vi "Preserve niDCPower Settings - PAE.vi"(7 "Action":enum16{"Reserve Settings", "Re-apply Settings"}(ring), 8 "error in":errorcluster, 10 "Active Channel":string="0", 11 "Resource Name":refnum<k15>="Dev1/0") -> (0 "error out":errorcluster, 1 "output cluster":T1, 2 "Active Channel":string="0", 3 "Resource Name":refnum<k15>)   [LabVIEW 2023]
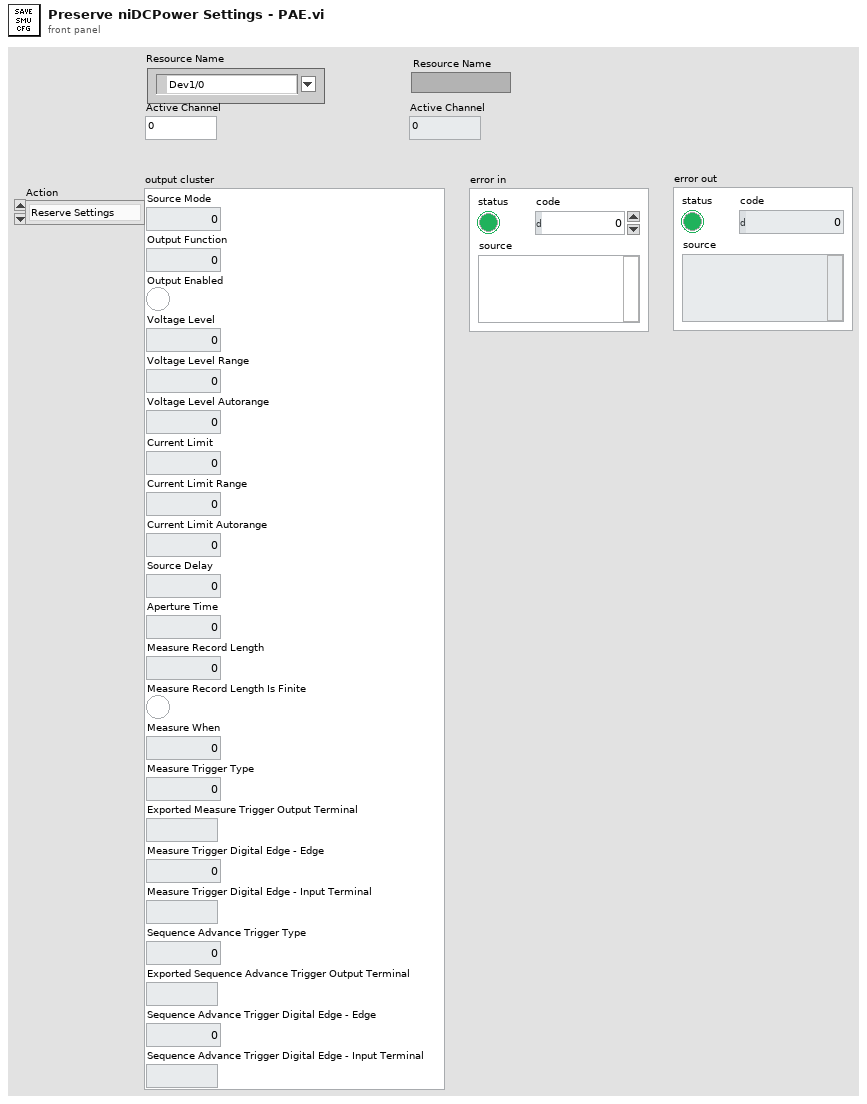
[diagram p1: front panel]
types:
  T1 = cluster{"Source Mode":i32, "Output Function":i32, "Output Enabled":bool, "Voltage Level":dbl, "Voltage Level Range":dbl, "Voltage Level Autorange":i32, "Current Limit":dbl, "Current Limit Range":dbl, "Current Limit Autorange":i32, "Source Delay":dbl, "Aperture Time":dbl, "Measure Record Length":i32, "Measure Record Length Is Finite":bool, "Measure When":i32, "Measure Trigger Type":i32, "Exported Measure Trigger Output Terminal":string, "Measure Trigger Digital Edge - Edge":i32, "Measure Trigger Digital Edge - Input Terminal":string, "Sequence Advance Trigger Type":i32, "Exported Sequence Advance Trigger Output Terminal":string, "Sequence Advance Trigger Digital Edge - Edge":i32, "Sequence Advance Trigger Digital Edge - Input Terminal":string}
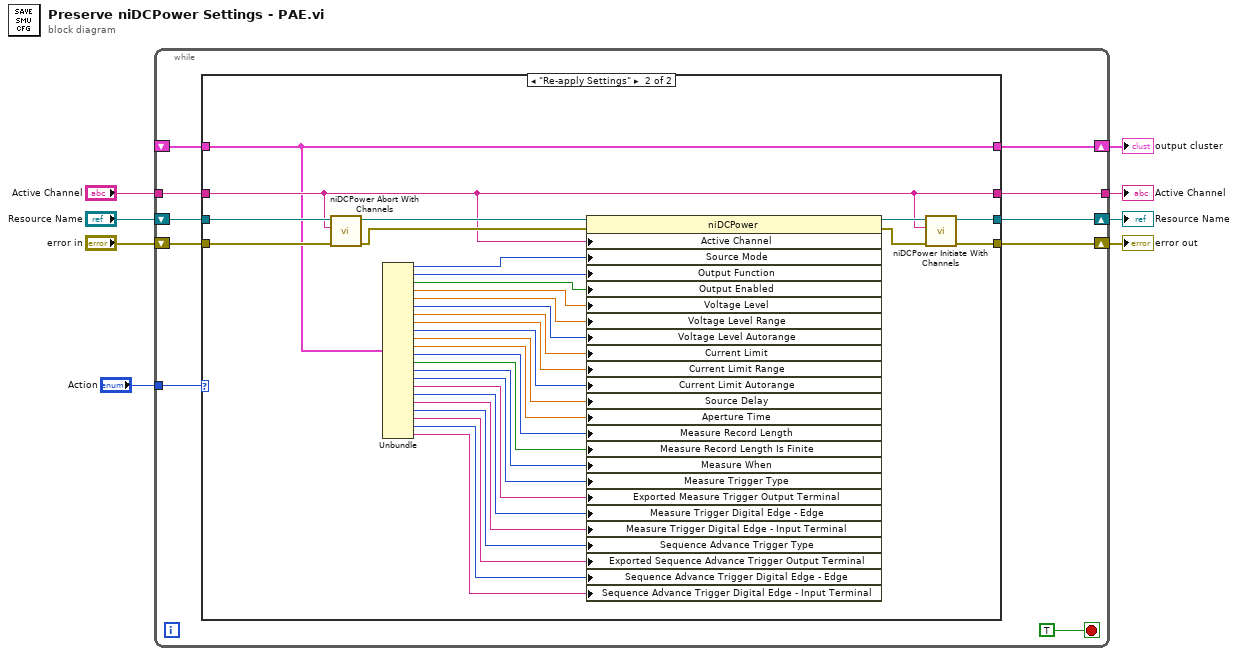
[diagram p0: block diagram]
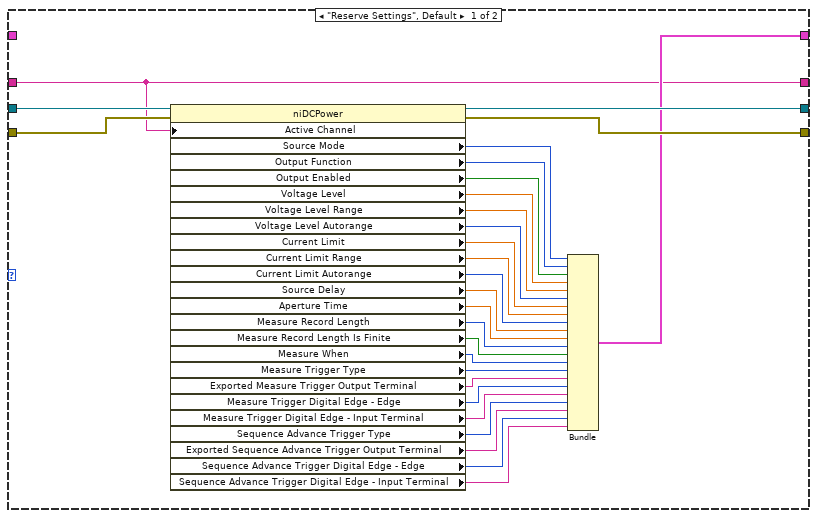
[diagram p2: hidden frame]
diagram:
  n1 = while {
    shift-right: [w16] -> w6
    shift-left: "Resource Name" -> [w18]
    shift-right: [w17] -> w7
    shift-left: "error in" -> [w15]
    shift-right: [w14] -> w1
    shift-left: _ -> [w12]
    tunnel: "Action" -> [w11]
    tunnel: "Active Channel" -> [w10]
    tunnel: [w9] -> w2
    stop <- TRUE stop-if-true
    n2 = case shown="\"Re-apply Settings\"" w11 {
      tunnel: w18 -> [w46 w56]
      tunnel: [w45 w51] -> w17
      tunnel: [w43 w49] -> w16
      tunnel: w15 -> [w21 w54]
      tunnel: [w20 w47] -> w14
      tunnel: w12 -> [_ w47]
      tunnel: w10 -> [w19 w48]
      tunnel: [w19 w48] -> w9
      frame "Reserve Settings", Default {
        n3 = property class="niDCPower"(reference=w46, error in=w21, "Active Channel"=w19) -> (reference out=w43:refnum<k15>, error out=w45:errorcluster, "Source Mode"=w44:i32, "Output Function"=w42:i32, "Output Enabled"=w41:bool, "Voltage Level"=w40:dbl, "Voltage Level Range"=w39:dbl, "Voltage Level Autorange"=w38:i32, "Current Limit"=w37:dbl, "Current Limit Range"=w36:dbl, "Current Limit Autorange"=w35:i32, "Source Delay"=w34:dbl, "Aperture Time"=w33:dbl, "Measure Record Length"=w32:i32, "Measure Record Length Is Finite"=w31:bool, "Measure When"=w30:i32, "Measure Trigger Type"=w29:i32, "Exported Measure Trigger Output Terminal"=w28:string, "Measure Trigger Digital Edge - Edge"=w27:i32, "Measure Trigger Digital Edge - Input Terminal"=w26:string, "Sequence Advance Trigger Type"=w25:i32, "Exported Sequence Advance Trigger Output Terminal"=w24:string, "Sequence Advance Trigger Digital Edge - Edge"=w23:i32, "Sequence Advance Trigger Digital Edge - Input Terminal"=w22:string)
        n4 = Bundle("Source Mode"=w44, "Output Function"=w42, "Output Enabled"=w41, "Voltage Level"=w40, "Voltage Level Range"=w39, "Voltage Level Autorange"=w38, "Current Limit"=w37, "Current Limit Range"=w36, "Current Limit Autorange"=w35, "Source Delay"=w34, "Aperture Time"=w33, "Measure Record Length"=w32, "Measure Record Length Is Finite"=w31, "Measure When"=w30, "Measure Trigger Type"=w29, "Exported Measure Trigger Output Terminal"=w28, "Measure Trigger Digital Edge - Edge"=w27, "Measure Trigger Digital Edge - Input Terminal"=w26, "Sequence Advance Trigger Type"=w25, "Exported Sequence Advance Trigger Output Terminal"=w24, "Sequence Advance Trigger Digital Edge - Edge"=w23, "Sequence Advance Trigger Digital Edge - Input Terminal"=w22) -> (w20:T1)  [unwired: 1 in]
      }
      frame "Re-apply Settings" {
        n5 = call <instrlib>:"niDCPower Abort With Channels.vi"("error in (no error)"=w54, "channel name"=w48, "instrument handle"=w56) -> ("error out"=w53:errorcluster, "instrument handle out"=w55:refnum<k15>)  [unwired: 7 in]
        n6 = Unbundle(w47) -> ("Source Mode"=w78:i32, "Output Function"=w77:i32, "Output Enabled"=w76:bool, "Voltage Level"=w75:dbl, "Voltage Level Range"=w74:dbl, "Voltage Level Autorange"=w73:i32, "Current Limit"=w72:dbl, "Current Limit Range"=w71:dbl, "Current Limit Autorange"=w70:i32, "Source Delay"=w69:dbl, "Aperture Time"=w68:dbl, "Measure Record Length"=w67:i32, "Measure Record Length Is Finite"=w66:bool, "Measure When"=w65:i32, "Measure Trigger Type"=w64:i32, "Exported Measure Trigger Output Terminal"=w63:string, "Measure Trigger Digital Edge - Edge"=w62:i32, "Measure Trigger Digital Edge - Input Terminal"=w61:string, "Sequence Advance Trigger Type"=w60:i32, "Exported Sequence Advance Trigger Output Terminal"=w59:string, "Sequence Advance Trigger Digital Edge - Edge"=w58:i32, "Sequence Advance Trigger Digital Edge - Input Terminal"=w57:string)
        n7 = property class="niDCPower"(reference=w55, error in=w53, "Active Channel"=w48, "Source Mode"=w78, "Output Function"=w77, "Output Enabled"=w76, "Voltage Level"=w75, "Voltage Level Range"=w74, "Voltage Level Autorange"=w73, "Current Limit"=w72, "Current Limit Range"=w71, "Current Limit Autorange"=w70, "Source Delay"=w69, "Aperture Time"=w68, "Measure Record Length"=w67, "Measure Record Length Is Finite"=w66, "Measure When"=w65, "Measure Trigger Type"=w64, "Exported Measure Trigger Output Terminal"=w63, "Measure Trigger Digital Edge - Edge"=w62, "Measure Trigger Digital Edge - Input Terminal"=w61, "Sequence Advance Trigger Type"=w60, "Exported Sequence Advance Trigger Output Terminal"=w59, "Sequence Advance Trigger Digital Edge - Edge"=w58, "Sequence Advance Trigger Digital Edge - Input Terminal"=w57) -> (reference out=w50:refnum<k15>, error out=w52:errorcluster)
        n8 = call <instrlib>:"niDCPower Initiate With Channels.vi"("error in (no error)"=w52, "channel name"=w48, "instrument handle"=w50) -> ("error out"=w51:errorcluster, "instrument handle out"=w49:refnum<k15>)  [unwired: 7 in]
      }
    }
  }
  "error out" <- w7
  "Resource Name" <- w6
  "output cluster" <- w1
  "Active Channel" <- w2
